vi "YKMW100 Send Message and Log.vi"(0 "VISA session":refnum<visa-resource-name>, 7 "Send Message (\"\")":string, 9 "Timeout (25000)":u32=3000, 11 "error in (no error)":errorcluster, 13 "Source (\"\")":string) -> (4 "dup VISA session":refnum<visa-resource-name>, 8 "Read Buffer":string, 15 "error out":errorcluster)   [LabVIEW 2023]
doc: "This VI sends the message. Then it returns the response."
panel:
  out "Debug Array":string[][](array[string])
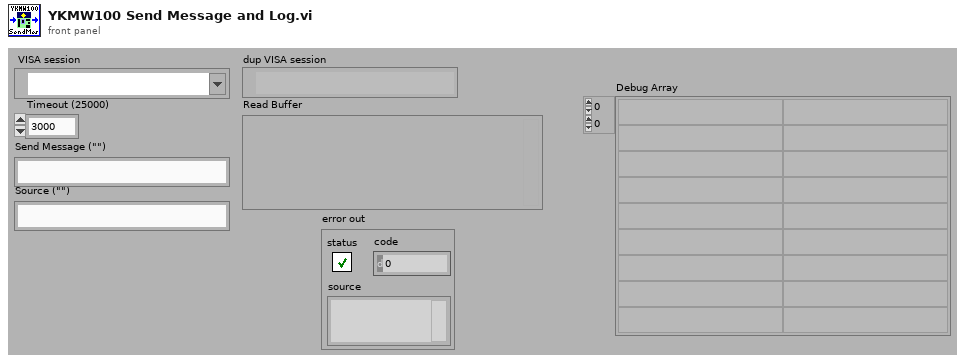
[diagram p1: front panel]
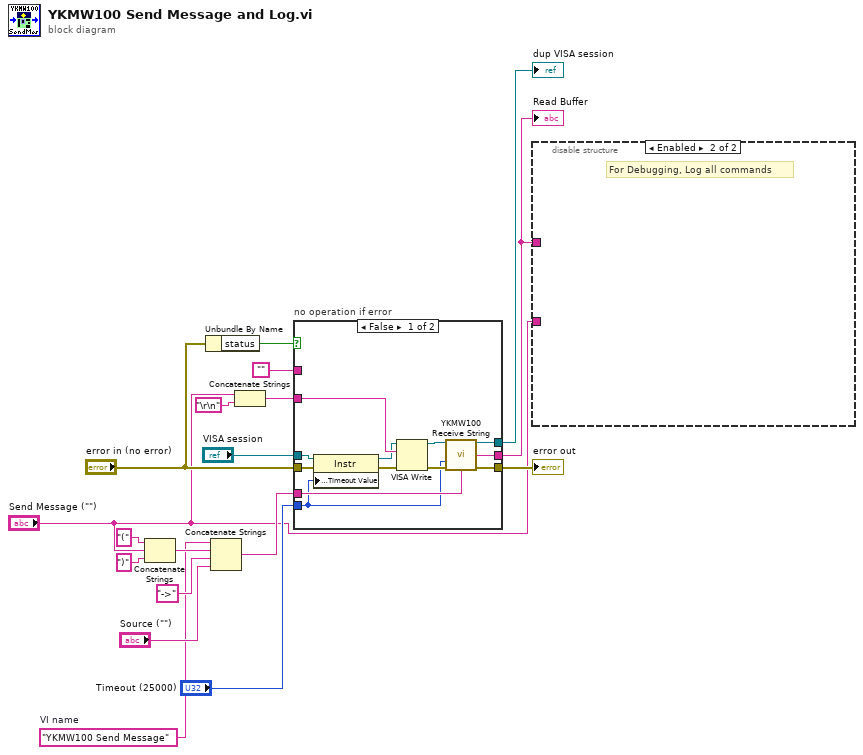
[diagram p0: block diagram]
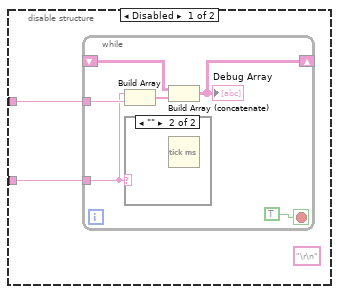
[diagram p2: hidden frame]
diagram:
  w7 = "YKMW100 Send Message"  # VI name
  n1 = Concatenate Strings("(", "Send Message (\"\")", ")") -> (w8:string)
  n2 = Unbundle By Name("error in (no error)") -> ("status"=w14:bool)
  n3 = Concatenate Strings(w7, w8, "->", "Source (\"\")") -> (w13:string)
  n4 = Concatenate Strings("Send Message (\"\")", "\r\n") -> (w17:string)
  n5 = case "no operation if error" shown="False" w14 {
    tunnel: "VISA session" -> [w27 w33]
    tunnel: w17 -> [w30 _]
    tunnel: [w24 w33] -> w6
    tunnel: [w22 w32] -> w18
    tunnel: "error in (no error)" -> [w29 w32]
    tunnel: w13 -> [w20 _]
    tunnel: "Timeout (25000)" -> [w19 _]
    tunnel: [w21 w31] -> w3
    tunnel: "" -> [_ w31]
    frame False {
      n6 = property class="Instr"(reference=w27, error in=w29, "General Settings:Timeout Value"=w19) -> (reference out=w26:refnum<visa-resource-name>, error out=w28:errorcluster)
      n7 = VISA Write(VISA resource name=w26, write buffer=w30, error in (no error)=w28) -> (VISA resource name out=w25:refnum<visa-resource-name>, error out=w23:errorcluster)  [unwired: 1 out]
      n8 = call "YKMW100 Receive String.vi"("VISA session"=w25, "Timeout (25000)"=w19, "error in (no error)"=w23, "Source (\"\")"=w20) -> ("dup VISA session"=w24:refnum<visa-resource-name>, "Read Buffer"=w21:string, "error out"=w22:errorcluster)  [unwired: 9 in]
    }
    frame True {
    }
  }
  "error out" <- w18
  "dup VISA session" <- w6
  "Read Buffer" <- w3
  n9 = disable-structure shown="Enabled" {
    disable-tunnel: w3 -> [w35 _]
    disable-tunnel: "Send Message (\"\")" -> [w34 _]
    frame Disabled {
      (unwired) "\r\n"
      n10 = while {
        tunnel: w35 -> [w40]
        tunnel: w34 -> [w39]
        shift-right: [w38] -> _
        shift-left: _ -> [w37]
        stop <- TRUE stop-if-true
        n11 = Build Array(w39, w40) -> (w36:string[])
        n12 = case shown="\"\"" w39 {
          frame "False", Default {
          }
          frame "" {
            n13 = Tick Count (ms)() -> ()  [unwired: 1 out]
          }
        }
        n14 = Build Array (concatenate)(w37, w36) -> (w38:string[][])
        "Debug Array" <- w38
      }
    }
    frame Enabled {
      # "For Debugging, Log all commands"
    }
  }
